vi "RP Lockin Continuous Sweeper.vi"(6 "Samples per read":i32=1024, 8 "Error In":errorcluster, 10 "Frequencies":dbl[](array[numeric]), 11 "connection ID":refnum<k5>) -> (0 "Error Out":errorcluster, 1 "Y":dbl[](array[numeric]), 2 "X":dbl[](array[numeric]), 3 "connection ID out":refnum<k5>, 4 "F":dbl[](array[numeric]))   [LabVIEW 2015]
panel:
  out "Input Fifo cnt 2":i32
  out "32bit integer":i32
  out "Output Fifo cnt":i32
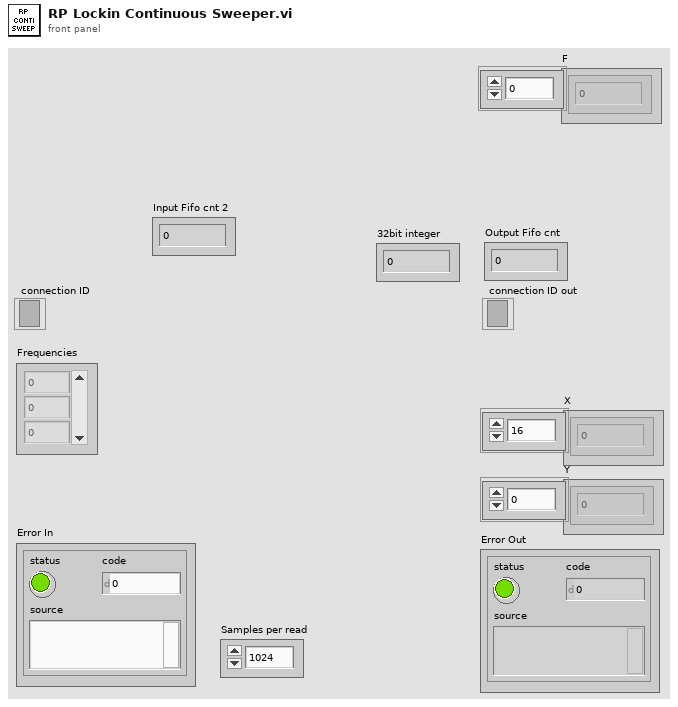
[diagram p1: front panel]
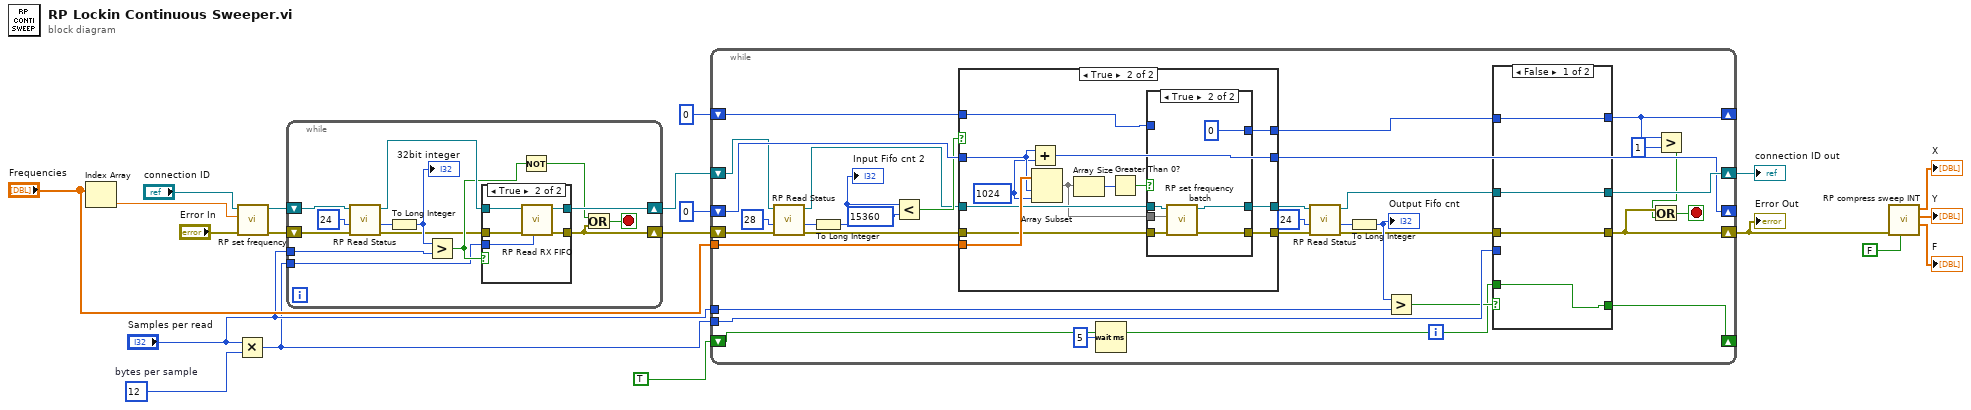
[diagram p0: block diagram]
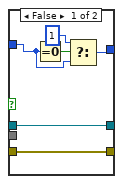
[diagram p4: hidden frame]
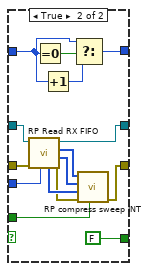
[diagram p5: hidden frame]
diagram:
  w15 = 12  # bytes per sample
  n1 = Index Array(array="Frequencies") -> (element=w19:dbl)  [unwired: 1 in]
  n2 = Multiply(x="Samples per read", y=w15) -> (x*y=w9:i32)
  n3 = call "RP set frequency.vi"("Error In"="Error In", "Frequency"=w19, "connection ID"="connection ID") -> ("Error Out"=w10:errorcluster, "connection ID out"=w12:refnum<k5>)  [unwired: 6 in, 1 out]
  n4 = while {
    tunnel: "Samples per read" -> [w31]
    shift-right: [w21] -> w8
    shift-left: w10 -> [w28]
    shift-right: [w26] -> w11
    shift-left: w12 -> [w27]
    tunnel: w9 -> [w25]
    stop <- w24 stop-if-true
    n5 = call "RP Read Status.vi"("Error In"=w28, "Status offset"=u64 24, "connection ID"=w27) -> ("Error Out"=w23:errorcluster, "Status response"=w32:u32, "connection ID out"=w30:refnum<k5>)  [unwired: 6 in]
    n6 = To Long Integer(number=w32) -> (32bit integer=w33:i32)
    "32bit integer" <- w33
    n7 = Greater?(x=w33, y=w31) -> (0:w29:bool)
    n8 = case shown="True" w29 {
      tunnel: w30 -> [w36 w41]
      tunnel: w23 -> [w35 w40]
      tunnel: [w35 w39] -> w21
      tunnel: [w36 w38] -> w26
      tunnel: w25 -> [_ w37]
      frame False {
      }
      frame True {
        n9 = call "RP Read RX FIFO.vi"("FIFO Bytes per read"=w37, "Error In"=w40, "connection ID"=w41) -> ("Error Out"=w39:errorcluster, "connection ID out"=w38:refnum<k5>)  [unwired: 4 in, 3 out]
      }
    }
    n10 = Not(x=w29) -> (.not. x?=w22:bool)
    n11 = Or(x=w22, y=w21) -> (x .or. y?=w24:bool)
  }
  n12 = while {
    shift-right: [w47] -> _
    shift-left: 0 -> [w49]
    tunnel: "Frequencies" -> [w74]
    tunnel: "Samples per read" -> [w73]
    tunnel: w9 -> [w72]
    shift-right: [w68] -> w5
    shift-left: w8 -> [w71]
    shift-right: [w70] -> w14
    shift-left: w11 -> [w50]
    shift-right: [w66] -> _
    shift-left: 0 -> [w67]
    shift-right: [w42] -> _
    shift-left: TRUE -> [w43]
    stop <- w69 stop-if-true
    n13 = call "RP Read Status.vi"("Error In"=w71, "Status offset"=u64 28, "connection ID"=w50) -> ("Error Out"=w54:errorcluster, "Status response"=w58:u32, "connection ID out"=w53:refnum<k5>)  [unwired: 6 in]
    n14 = To Long Integer(number=w58) -> (32bit integer=w59:i32)
    "Input Fifo cnt 2" <- w59
    n15 = Less?(x=w59, y=15360) -> (x < y?=w55:bool)
    n16 = case shown="True" w55 {
      tunnel: w67 -> [w78 w90]
      tunnel: w74 -> [_ w91]
      tunnel: [w78 w88] -> w66
      tunnel: w54 -> [w76 w86]
      tunnel: w53 -> [w77 w85]
      tunnel: [w77 w84] -> w52
      tunnel: [w76 w83] -> w51
      tunnel: w49 -> [w75 w80]
      tunnel: [w75 w79] -> w48
      frame False {
      }
      frame True {
        w89 = 1024
        n17 = Add(x=w90, y=w89) -> (x+y=w88:i32)
        n18 = Array Subset(array=w91, index=w90, length=w89) -> (w82:dbl[])
        n19 = Array Size(array=w82) -> (size(s)=w87:i32)
        n20 = Greater Than 0?(x=w87) -> (x > 0?=w81:bool)
        n21 = case shown="True" w81 {
          tunnel: w86 -> [w97 w103]
          tunnel: w85 -> [w96 w102]
          tunnel: [w96 w101] -> w84
          tunnel: [w97 w100] -> w83
          tunnel: w82 -> [_ w99]
          tunnel: w80 -> [w92 _]
          tunnel: [w93 0] -> w79
          frame False {
            n22 = Equal To 0?(x=w92) -> (x = 0?=w95:bool)
            n23 = Select(t=1, s=w95, f=w92) -> (s? t:f=w93:i32)
          }
          frame True {
            n24 = call "RP set frequency batch.vi"("Error In"=w103, "Frequency"=w99, "connection ID"=w102) -> ("Error Out"=w100:errorcluster, "connection ID out"=w101:refnum<k5>)  [unwired: 7 in]
          }
        }
      }
    }
    n25 = Wait (ms)(milliseconds to wait=u32 5) -> ()  [unwired: 1 out]
    n26 = call "RP Read Status.vi"("Error In"=w51, "Status offset"=u64 24, "connection ID"=w52) -> ("Error Out"=w60:errorcluster, "Status response"=w64:u32, "connection ID out"=w61:refnum<k5>)  [unwired: 6 in]
    n27 = To Long Integer(number=w64) -> (32bit integer=w63:i32)
    "Output Fifo cnt" <- w63
    n28 = Greater?(x=w63, y=w73) -> (0:w62:bool)
    n29 = case shown="False" w62 {
      tunnel: w72 -> [_ w122]
      tunnel: w61 -> [w106 w121]
      tunnel: w60 -> [w107 w120]
      tunnel: [w107 w113] -> w68
      tunnel: [w106 w119] -> w70
      tunnel: w43 -> [w104 w115]
      tunnel: w48 -> [w105 w110]
      tunnel: [w105 w111] -> w47
      tunnel: [w104 FALSE] -> w42
      frame False {
      }
      frame True {
        n30 = call "RP Read RX FIFO.vi"("FIFO Bytes per read"=w122, "Error In"=w120, "connection ID"=w121) -> ("Error Out"=w114:errorcluster, "Y"=w116:i32[], "X"=w118:i32[], "connection ID out"=w119:refnum<k5>, "F"=w117:i32[])  [unwired: 4 in]
        n31 = Equal To 0?(x=w110) -> (x = 0?=w112:bool)
        n32 = Increment(x=w110) -> (x+1=w109:i32)
        n33 = Select(t=w110, s=w112, f=w109) -> (s? t:f=w111:i32)
        n34 = call "RP compress sweep INT.vi"("First call?"=w115, "Error In"=w114, "F"=w117, "Y"=w116, "X"=w118) -> ("Error Out"=w113:errorcluster)  [unwired: 3 in, 3 out]
      }
    }
    n35 = Greater?(x=w47, y=1) -> (0:w45:bool)
    n36 = Or(x=w68, y=w45) -> (x .or. y?=w69:bool)
  }
  "connection ID out" <- w14
  "Error Out" <- w5
  n37 = call "RP compress sweep INT.vi"("First call?"=FALSE, "Error In"=w5) -> ("F out"=→"F":dbl[], "Y out"=→"Y":dbl[], "X out"=→"X":dbl[])  [unwired: 6 in, 1 out]
